vi "Parse Data Filename (CFTS).vi"(0 "Path":path) -> (3 "Folder":path, 4 "User ID":string, 6 "Animal number":i32, 8 "Data type":string)   [LabVIEW 2020]
uses:
  <vilib>/regexp/Match Regular Expression.xnode
panel:
  out "Run number":i32
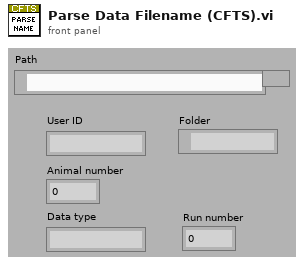
[diagram p1: front panel]
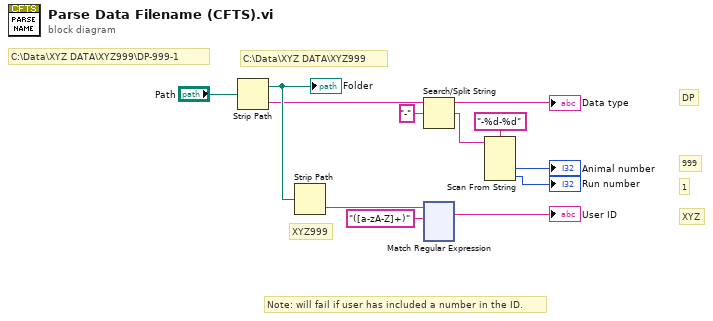
[diagram p0: block diagram]
diagram:
  # "Note: will fail if user has included a number in the ID."
  # "1"
  # "999"
  # "DP"
  # "XYZ"
  # "XYZ999"
  # "C:\\Data\\XYZ DATA\\XYZ999"
  # "C:\\Data\\XYZ DATA\\XYZ999\\DP-999-1"
  n1 = Strip Path(path="Path") -> (stripped path=w8:path, name=w7:string)
  "Folder" <- w8
  n2 = Strip Path(path=w8) -> (name=w11:string)  [unwired: 1 out]
  n3 = Search/Split String(string=w7, search string/char (-)="-") -> (substring before match=→"Data type":string, match + rest of string=w4:string)  [unwired: 1 in, 1 out]
  n4 = xnode "Match Regular Expression"("input string"=w11, "regular expression"="([a-zA-Z]+)") -> ("whole match"=→"User ID":string)  [unwired: 4 in, 4 out]
  n5 = Scan From String(format string="-%d-%d", input string=w4) -> (output 1=→"Animal number":i32, output 2=→"Run number":i32)  [unwired: 4 in, 3 out]
